vi "Autonomous Independent.vi"   [LabVIEW 2020]
doc: "This VI is called when autonomous begins, and will automatically be terminated when autonomous ends. You can carry out timed or sensor driven robot movement independently without needing to return to the caller."
uses:
  <vilib>/Rock Robotics/Network Tables/NT Read String.vi
  Robot Global Data.vi
panel:
  # "Be sure to right-click and choose Data Operations>>Make Current Value default if you want to save the array values with the VI"
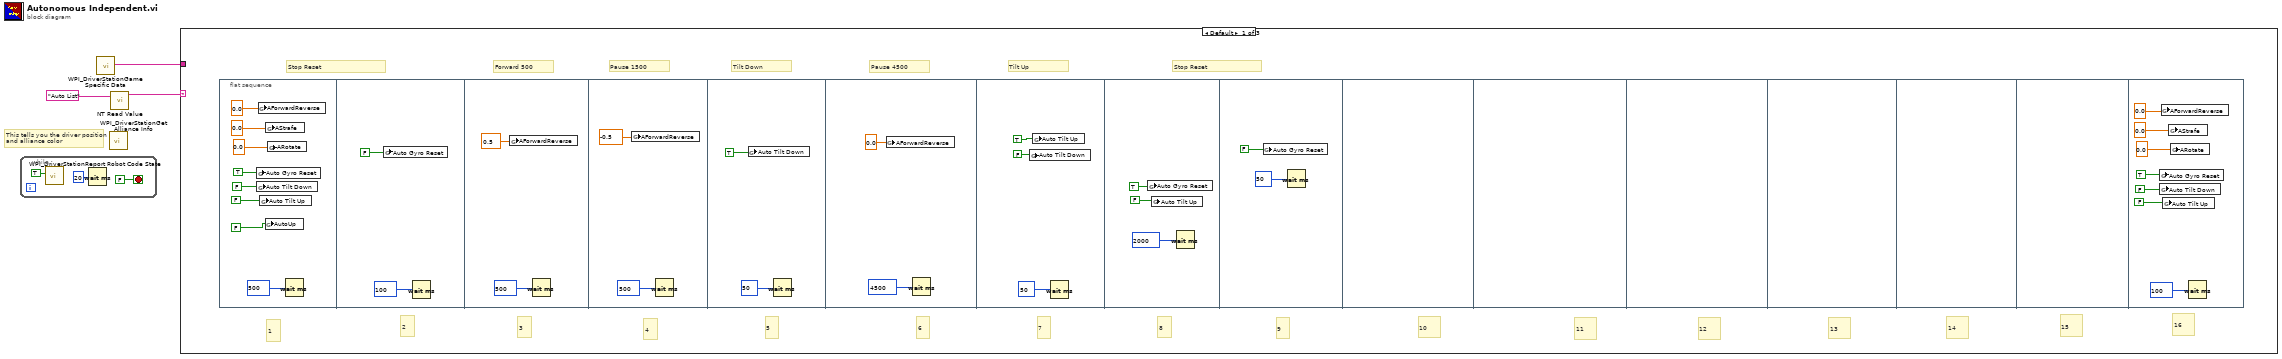
[diagram p0: block diagram]
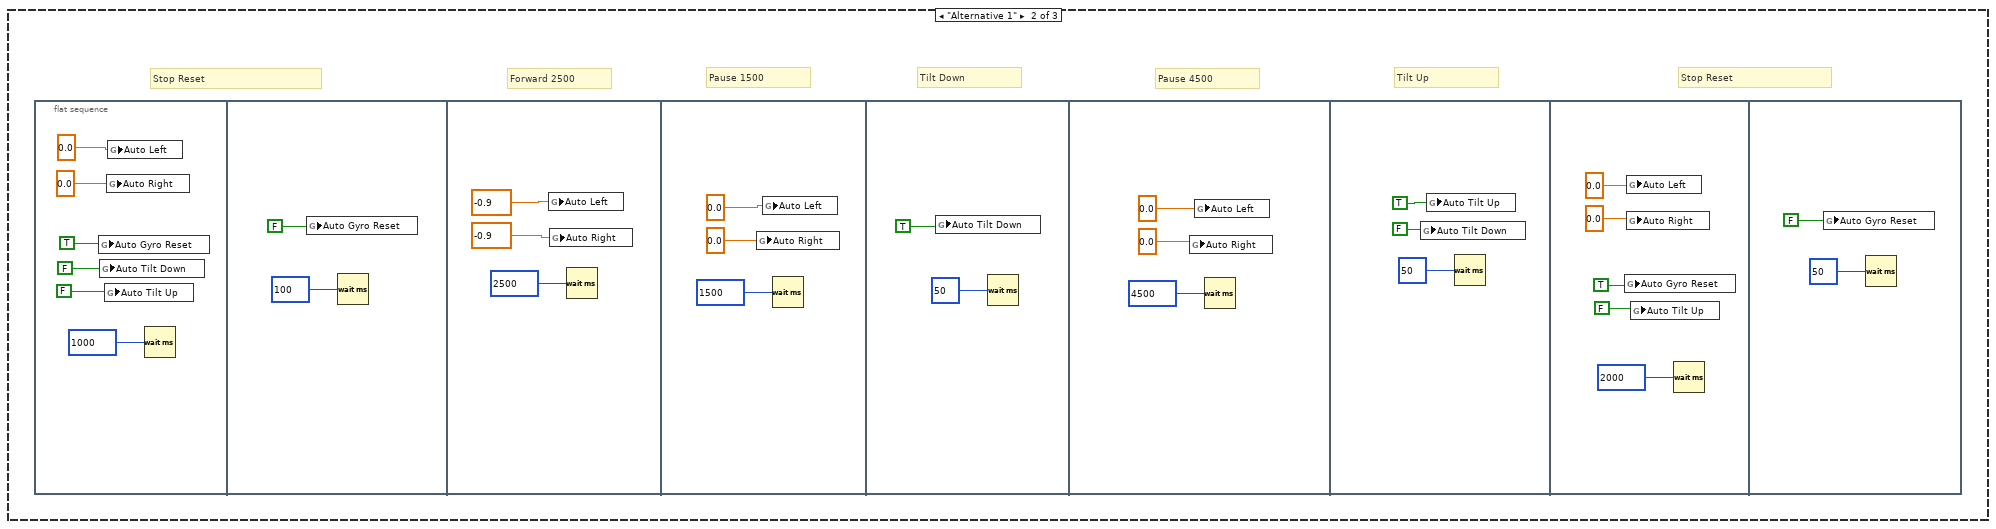
[diagram p2: hidden frame]
diagram:
  # "This tells you the driver position\nand alliance color"
  n1 = while {
    stop <- FALSE stop-if-true
    n2 = call <vilib>:"WPI_DriverStationReport Robot Code State.vi"("Autonomous"=TRUE) -> ()  [unwired: 10 in, 1 out]
    n3 = Wait (ms)(milliseconds to wait=u32 20) -> ()  [unwired: 1 out]
  }
  n4 = call <vilib>:"WPI_DriverStationGame Specific Data.vi"() -> ("Game Specific Data"=w1:string)  [unwired: 11 in]
  n5 = call <vilib>:"WPI_DriverStationGet Alliance Info.vi"() -> ()  [unwired: 12 out]
  n6 = call-poly <vilib>:"NT Read Value.vi"("Name"="Auto List") -> ("String"=w2:string)  [unwired: 9 in, 1 out]
  n7 = case shown="Default" w2 {
    tunnel: w1 -> [_ _ _]
    frame Default {
      # "16"
      # "15"
      # "14"
      # "13"
      # "12"
      # "11"
      # "10"
      # "9"
      # "8"
      # "7"
      # "6"
      # "5"
      # "4"
      # "3"
      # "2"
      # "1"
      # "Stop Reset"
      # "Tilt Up"
      # "Pause 4500"
      # "Tilt Down"
      # "Pause 1500"
      # "Forward 500"
      # "Stop Reset"
      n8 = flat-sequence {
        frame #0 {
          n9 = global write "Robot Global Data.vi" "Auto Gyro Reset"(TRUE) -> ()
          n10 = global write "Robot Global Data.vi" "Auto Tilt Down"(FALSE) -> ()
          n11 = global write "Robot Global Data.vi" "AForwardReverse"(0.0 ("Autonomous Shooter")) -> ()
          n12 = global write "Robot Global Data.vi" "Auto Tilt Up"(FALSE) -> ()
          n13 = global write "Robot Global Data.vi" "AutoUp"(FALSE) -> ()
          n14 = global write "Robot Global Data.vi" "AStrafe"(0.0 ("Autonomous Shooter")) -> ()
          n15 = global write "Robot Global Data.vi" "ARotate"(0.0 ("Autonomous Shooter")) -> ()
          n16 = Wait (ms)(milliseconds to wait=u32 500) -> ()  [unwired: 1 out]
        }
        frame #1 {
          n17 = global write "Robot Global Data.vi" "Auto Gyro Reset"(FALSE) -> ()
          n18 = Wait (ms)(milliseconds to wait=u32 100) -> ()  [unwired: 1 out]
        }
        frame #2 {
          n19 = global write "Robot Global Data.vi" "AForwardReverse"(0.5 ("Autonomous Shooter")) -> ()
          n20 = Wait (ms)(milliseconds to wait=u32 500) -> ()  [unwired: 1 out]
        }
        frame #3 {
          n21 = global write "Robot Global Data.vi" "AForwardReverse"(-0.5 ("Autonomous Shooter")) -> ()
          n22 = Wait (ms)(milliseconds to wait=u32 500) -> ()  [unwired: 1 out]
        }
        frame #4 {
          n23 = global write "Robot Global Data.vi" "Auto Tilt Down"(TRUE) -> ()
          n24 = Wait (ms)(milliseconds to wait=u32 50) -> ()  [unwired: 1 out]
        }
        frame #5 {
          n25 = global write "Robot Global Data.vi" "AForwardReverse"(0.0 ("Autonomous Shooter")) -> ()
          n26 = Wait (ms)(milliseconds to wait=u32 4500) -> ()  [unwired: 1 out]
        }
        frame #6 {
          n27 = global write "Robot Global Data.vi" "Auto Tilt Down"(FALSE) -> ()
          n28 = global write "Robot Global Data.vi" "Auto Tilt Up"(TRUE) -> ()
          n29 = Wait (ms)(milliseconds to wait=u32 50) -> ()  [unwired: 1 out]
        }
        frame #7 {
          n30 = global write "Robot Global Data.vi" "Auto Gyro Reset"(TRUE) -> ()
          n31 = global write "Robot Global Data.vi" "Auto Tilt Up"(FALSE) -> ()
          n32 = Wait (ms)(milliseconds to wait=u32 2000) -> ()  [unwired: 1 out]
        }
        frame #8 {
          n33 = global write "Robot Global Data.vi" "Auto Gyro Reset"(FALSE) -> ()
          n34 = Wait (ms)(milliseconds to wait=u32 50) -> ()  [unwired: 1 out]
        }
        frame #9 {
        }
        frame #10 {
        }
        frame #11 {
        }
        frame #12 {
        }
        frame #13 {
        }
        frame #14 {
        }
        frame #15 {
          n35 = global write "Robot Global Data.vi" "Auto Gyro Reset"(TRUE) -> ()
          n36 = global write "Robot Global Data.vi" "Auto Tilt Down"(FALSE) -> ()
          n37 = global write "Robot Global Data.vi" "AForwardReverse"(0.0 ("Autonomous Shooter")) -> ()
          n38 = global write "Robot Global Data.vi" "Auto Tilt Up"(FALSE) -> ()
          n39 = global write "Robot Global Data.vi" "AStrafe"(0.0 ("Autonomous Shooter")) -> ()
          n40 = global write "Robot Global Data.vi" "ARotate"(0.0 ("Autonomous Shooter")) -> ()
          n41 = Wait (ms)(milliseconds to wait=u32 100) -> ()  [unwired: 1 out]
        }
      }
    }
    frame "Alternative 1" {
      # "Stop Reset"
      # "Tilt Up"
      # "Pause 4500"
      # "Tilt Down"
      # "Pause 1500"
      # "Forward 2500"
      # "Stop Reset"
      n42 = flat-sequence {
        frame #0 {
          n43 = global write "Robot Global Data.vi" "Auto Gyro Reset"(TRUE) -> ()
          n44 = global write "Robot Global Data.vi" "Auto Tilt Down"(FALSE) -> ()
          n45 = global write "Robot Global Data.vi" "Auto Tilt Up"(FALSE) -> ()
          n46 = global write "Robot Global Data.vi" "Auto Right"(0.0 ("Autonomous Shooter")) -> ()
          n47 = global write "Robot Global Data.vi" "Auto Left"(0.0 ("Autonomous Shooter")) -> ()
          n48 = Wait (ms)(milliseconds to wait=u32 1000) -> ()  [unwired: 1 out]
        }
        frame #1 {
          n49 = global write "Robot Global Data.vi" "Auto Gyro Reset"(FALSE) -> ()
          n50 = Wait (ms)(milliseconds to wait=u32 100) -> ()  [unwired: 1 out]
        }
        frame #2 {
          n51 = global write "Robot Global Data.vi" "Auto Left"(-0.9 ("Autonomous Shooter")) -> ()
          n52 = global write "Robot Global Data.vi" "Auto Right"(-0.9 ("Autonomous Shooter")) -> ()
          n53 = Wait (ms)(milliseconds to wait=u32 2500) -> ()  [unwired: 1 out]
        }
        frame #3 {
          n54 = global write "Robot Global Data.vi" "Auto Right"(0.0 ("Autonomous Shooter")) -> ()
          n55 = global write "Robot Global Data.vi" "Auto Left"(0.0 ("Autonomous Shooter")) -> ()
          n56 = Wait (ms)(milliseconds to wait=u32 1500) -> ()  [unwired: 1 out]
        }
        frame #4 {
          n57 = global write "Robot Global Data.vi" "Auto Tilt Down"(TRUE) -> ()
          n58 = Wait (ms)(milliseconds to wait=u32 50) -> ()  [unwired: 1 out]
        }
        frame #5 {
          n59 = global write "Robot Global Data.vi" "Auto Right"(0.0 ("Autonomous Shooter")) -> ()
          n60 = global write "Robot Global Data.vi" "Auto Left"(0.0 ("Autonomous Shooter")) -> ()
          n61 = Wait (ms)(milliseconds to wait=u32 4500) -> ()  [unwired: 1 out]
        }
        frame #6 {
          n62 = global write "Robot Global Data.vi" "Auto Tilt Down"(FALSE) -> ()
          n63 = global write "Robot Global Data.vi" "Auto Tilt Up"(TRUE) -> ()
          n64 = Wait (ms)(milliseconds to wait=u32 50) -> ()  [unwired: 1 out]
        }
        frame #7 {
          n65 = global write "Robot Global Data.vi" "Auto Gyro Reset"(TRUE) -> ()
          n66 = global write "Robot Global Data.vi" "Auto Left"(0.0 ("Autonomous Shooter")) -> ()
          n67 = global write "Robot Global Data.vi" "Auto Right"(0.0 ("Autonomous Shooter")) -> ()
          n68 = global write "Robot Global Data.vi" "Auto Tilt Up"(FALSE) -> ()
          n69 = Wait (ms)(milliseconds to wait=u32 2000) -> ()  [unwired: 1 out]
        }
        frame #8 {
          n70 = global write "Robot Global Data.vi" "Auto Gyro Reset"(FALSE) -> ()
          n71 = Wait (ms)(milliseconds to wait=u32 50) -> ()  [unwired: 1 out]
        }
      }
    }
    frame "Alternative 2" {
    }
  }
